vi "Offset Locking and Active Slave Locking v3.1.vi"() -> ()   [LabVIEW 2018]
uses:
  <vilib>/Utility/error.llb/DialogType.ctl
  <vilib>/Analysis/1siggen.llb/Ramp Pattern by Samples.vi
  <vilib>/measure/mamon.llb/Waveform Peak Detection for 1 Chan.vi
  <vilib>/addons/control/pid/pid.llb/PID Advanced (DBL).vi
  <vilib>/measure/NI_MAPro.lvlib
  <vilib>/addons/control/pid/NI_PID_pid.lvlib
  <vilib>/Analysis/NI_AALBase.lvlib
  <vilib>/measure/NI_MABase.lvlib
panel:
  out "Master-Slave Peak Height":dbl
  in  "Locked Peak Height Min":dbl
  in  "Active Slave Lock On":bool
  in  "Slave Current Adjust":dbl
  out "Target \nPeak":dbl
  out "Calibration\n Peaks":dbl[](array[numeric])
  in  "Minimum \namplitude\nfor Calibration":dbl=2.1 format="%#_13g V"
  in  "width":i32=1000
  in  "start":dbl format="%0.2f"
  in  "end":dbl=1.0 format="%0.2f"
  in  "samples":i32=128
  in  "Waveform Test?":bool
  in  "reset signal":bool
  in  "phase":dbl format="%.2p"
  out "Chirp Rate":dbl format="%#_g GHz/ms"
  out "Single Mode?":bool
  out "# of Peaks found when Chirping?":i32
  in  "Minimum amplitude for Slave":dbl=0.15 format="%.2p"
  in  "Minimum \namplitude\nfor peaks":dbl=1.2 format="%#_13g V"
  in  "PZT Voltage to \nFrequency Conversion":dbl=-1.41655 format="%#_g V/GHz"
  out "PZT Chirp Output":waveform(dbl)(graph)
  in  "offset":dbl format="%0.2p V"
  in  "Sampling Info":cluster{"Fs":dbl, "#s":dbl}={"Fs"=10000.0, "#s"=100.0} {"Fs" format="%.2p"}
  in  "frequency":dbl=10.0 format="%0.2p Hz"
  in  "Chirp Amplitude":dbl=1.5 format="%0.2p GHz"
  in  "Run Chirp Program?":bool
  out "Run Time (min)":dbl
  out "standard deviation":dbl format="%0.3e"
  out "# found":i32
  out "Offset":dbl(graph)
  in  "Manual PZT Control":dbl format="%#_g V"
  in  "Engage PZT PID?":bool
  out "Offset (GHz)":dbl format="%#_4g"
  in  "# of Shots for Averaging":i32=100
  in  "Name Convention":string="Chirp Offset Lock Log"
  in  "Save Directory":path=path "C:/Users/LabUser/Google Drive/Measurements/04-2018"
  out "Enough\n peaks?":bool
  out "PZT Output":dbl(graph)
  in  "PID Gains":T1={"proportional gain (Kc)"=-1.0, "integral time (Ti, min)"=0.01, "derivative time (Td, min)"=0.0} {"derivative time (Td, min)" format="%.3f"; "integral time (Ti, min)" format="%.3f"; "proportional gain (Kc)" format="%.3f"}
  out "dt out (s)":dbl format="%.3f"
  in  "Frequency Offset Setpoint (GHz)":dbl=4.0 format="%.3f"
  out "GHz/sec":dbl
  out "dt":dbl format="%#_4g"
  out "Locations":dbl[](array[numeric]) format="%.2p"
  out "Amplitudes":dbl[](array[numeric]) format="%.2p"
  out "2nd Derivatives":dbl[](array[numeric]) format="%.2p"
  out "10 GHz FPI":dynamicdata(graph)
  in  "Stop":bool
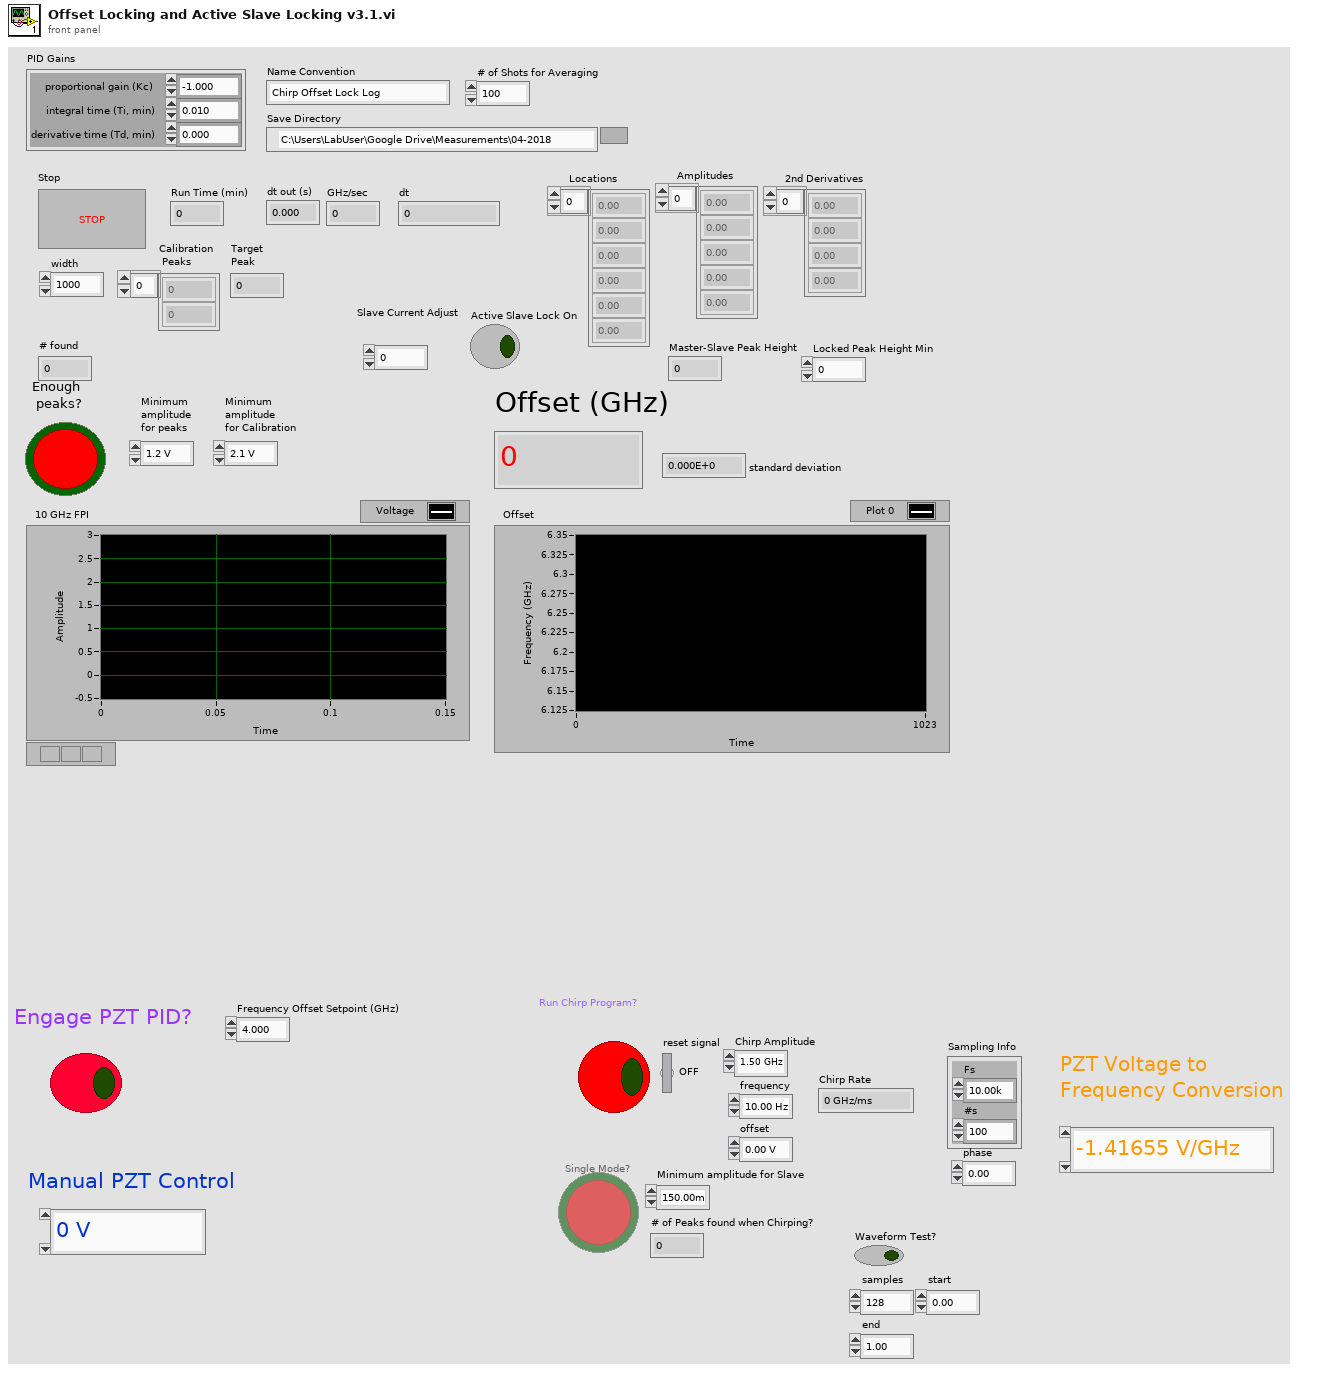
[diagram p1: front panel]
types:
  T1 = cluster{"proportional gain (Kc)":dbl, "integral time (Ti, min)":dbl, "derivative time (Td, min)":dbl}
  T2 = enum8{"Enabled", "Disabled", "Disabled and Grayed Out"}
  T3 = typedef "DialogType.ctl" = u16
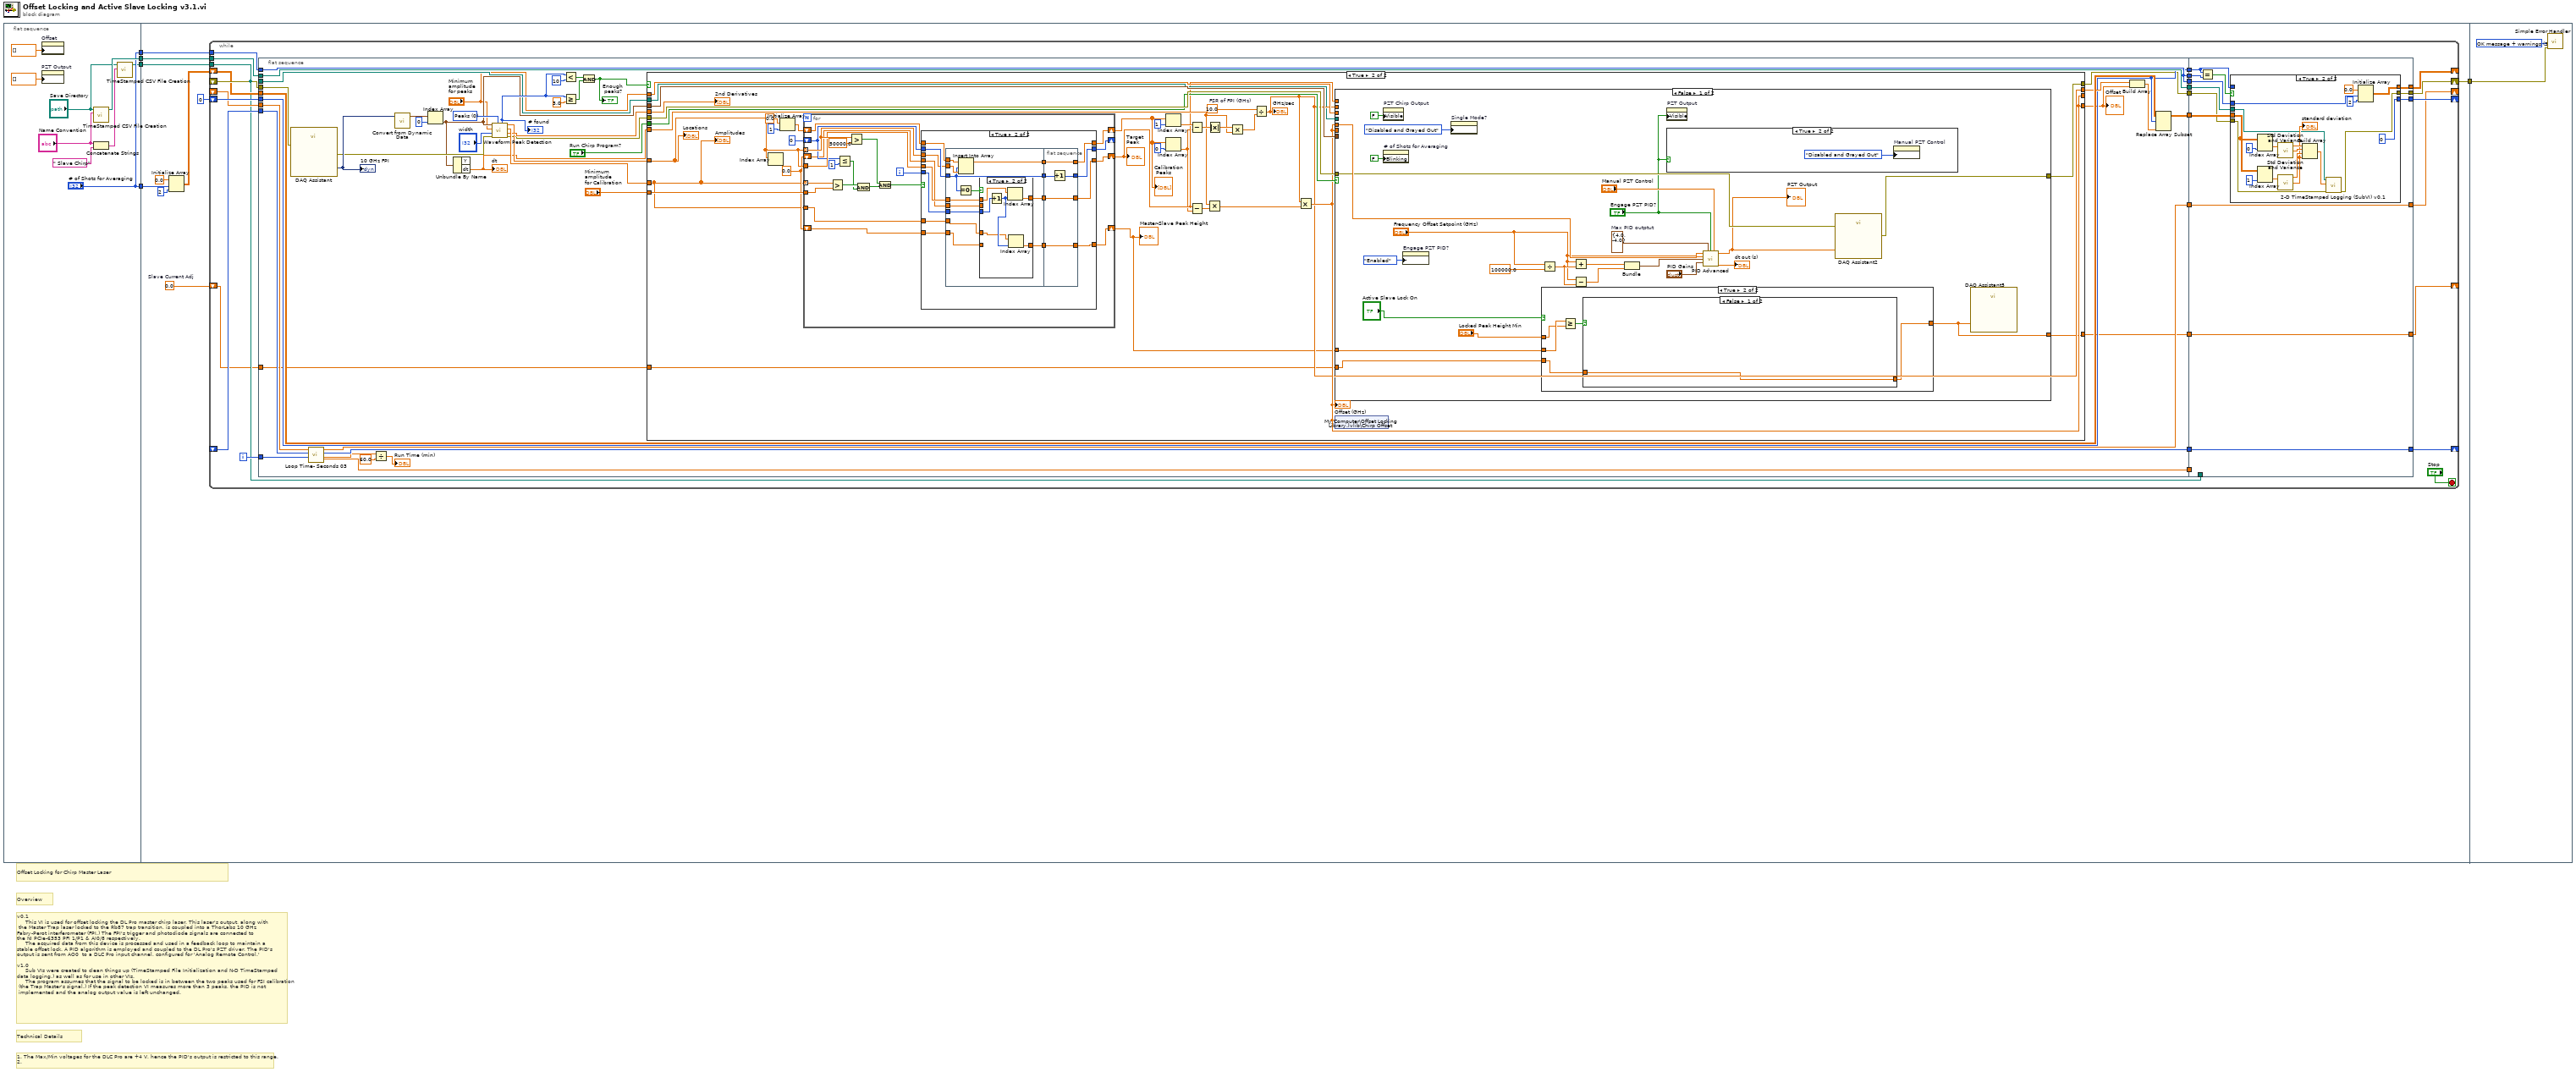
[diagram p0: block diagram]
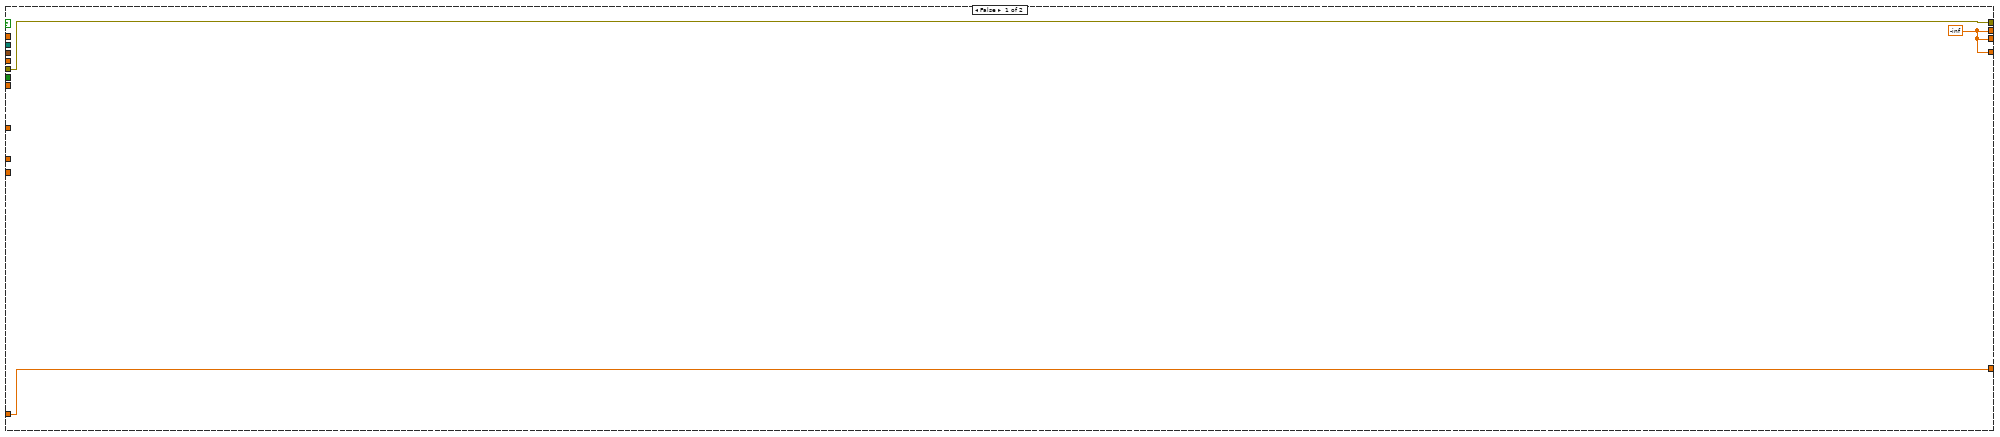
[diagram p2: hidden frame]
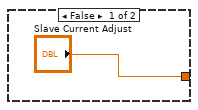
[diagram p5: hidden frame]
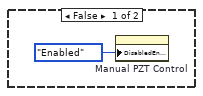
[diagram p7: hidden frame]
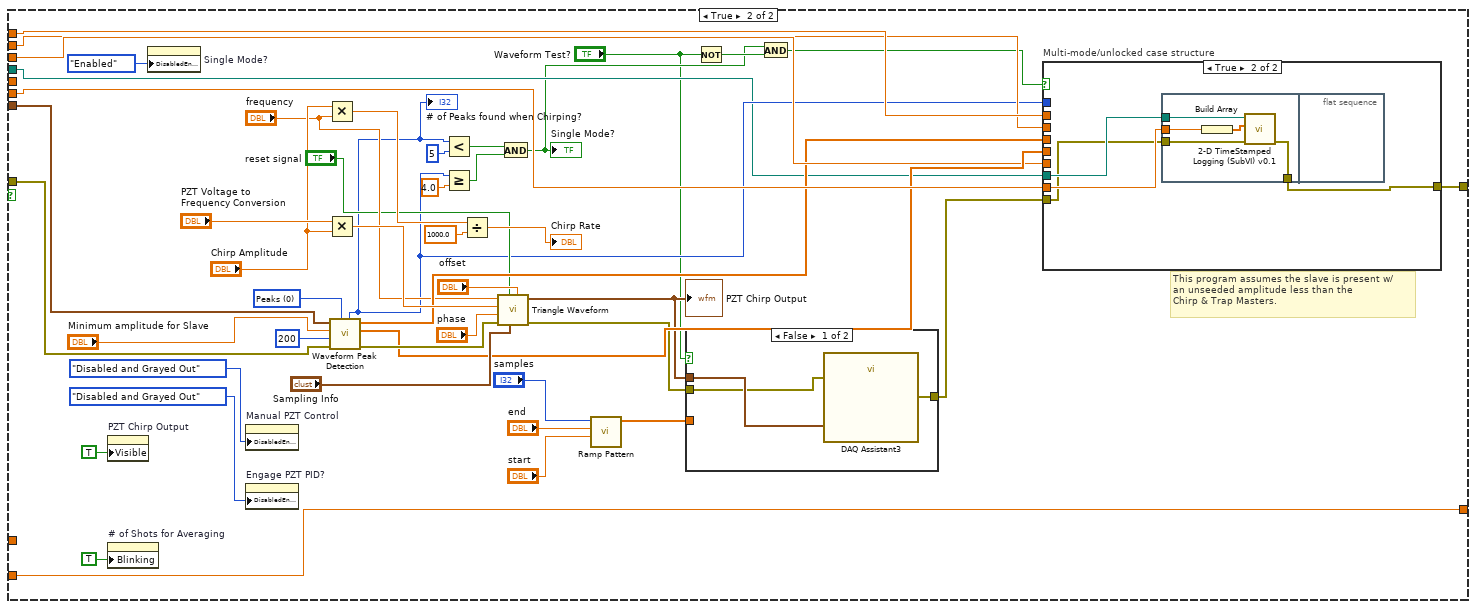
[diagram p8: hidden frame]
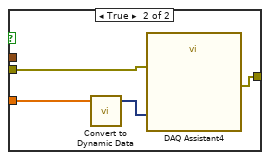
[diagram p9: hidden frame]
diagram:
  # "1. The Max/Min voltages for the DLC Pro are +4 V, hence the PID's output is restricted to this range.\n2."
  # "Technical Details"
  # "v0.1\n     This VI is used for offset locking the DL Pro master chirp laser. This laser's output, along with\n the Master Trap laser locked to the Rb87 trap transition, is coupled into a ThorLabs 10 GHz \nFabry-Perot interferometer (FPI.) The FPI's trigger and photodiode signals are connected to \nthe NI PCIe-6353 PFI 1/P1 & AI0/8 respectively. \n     The acquired data from this device is processed and used in a feedback loop to maintain a \nstable offset lock. A PID algorithm is employed and coupled to the DL Pro's PZT driver. The PID's\noutput is sent from AO0  to a DLC Pro input channel, configured for 'Analog Remote Control.'\n\nv1.0\n     Sub VIs were created to clean things up (TimeStamped File Initialization and N-D TimeStamped \ndata logging,) as well as for use in other VIs.\n     The program assumes that the signal to be locked is in between the two peaks used for FSI calibration\n (the Trap Master's signal.) If the peak detection VI measures more than 3 peaks, the PID is not\n implemented and the analog output value is left unchanged."
  # "Overview"
  # "Offset Locking for Chirp Master Laser"
  n1 = flat-sequence {
    tunnel: [w14] -> w5
    tunnel: ["# of Shots for Averaging"] -> w3
    tunnel: ["# of Shots for Averaging"] -> w2
    tunnel: [w6] -> w1
    tunnel: w5 -> [w24]
    tunnel: [w23] -> w4
    tunnel: w3 -> [w21]
    tunnel: w2 -> [w18]
    tunnel: w1 -> [w16]
    tunnel: w4 -> [w334]
    frame #0 {
      n2 = property on="Offset" class="WFChart (strict)"("History Data"=dbl[] []) -> ()  [unwired: 2 in, 2 out]
      n3 = property on="PZT Output" class="WFChart (strict)"("History Data"=dbl[] []) -> ()  [unwired: 2 in, 2 out]
      n4 = call "TimeStamped CSV File Creation.vi"("Name Convention"="Name Convention", "Save Directory"="Save Directory") -> ("path"=w14:path)  [unwired: 8 in, 1 out]
      n5 = Concatenate Strings("Name Convention", " Slave Chirp" ("string")) -> (w8:string)
      n6 = call "TimeStamped CSV File Creation.vi"("Name Convention"=w8, "Save Directory"="Save Directory") -> ("path"=w6:path)  [unwired: 8 in, 1 out]
    }
    frame #1 {
      w15 = 0.0  # Slave Current Adj
      n7 = Initialize Array(0.0 ("element"), w18, 2 ("dimension size")) -> (w20:dbl[][])
      n8 = while {
        shift-right: [w39] -> w23
        shift-left: _ -> [w50]
        tunnel: w24 -> [w48]
        shift-right: [w37] -> _
        shift-left: 0 -> [w46]
        tunnel: w21 -> [w44]
        shift-right: [w38] -> _
        shift-left: w20 -> [w41]
        shift-right: [w35] -> _
        shift-left: _ -> [w32]
        shift-right: [w33] -> _
        shift-left: _ -> [w31]
        tunnel: w16 -> [w28]
        shift-right: [w25] -> _
        shift-left: w15 -> [w27]
        i -> [w30]
        stop <- "Stop" stop-if-true
        n9 = flat-sequence {
          tunnel: w50 -> [w84]
          tunnel: [w60] -> w49
          tunnel: w48 -> [w82]
          tunnel: [w82] -> w47
          tunnel: w46 -> [w76]
          tunnel: [w76] -> w45
          tunnel: w44 -> [w77]
          tunnel: [w77] -> w43
          tunnel: [w81] -> w42
          tunnel: w41 -> [w80]
          tunnel: [w77] -> w40
          tunnel: [w75] -> w36
          tunnel: [w74] -> w34
          tunnel: w32 -> [w73]
          tunnel: w31 -> [w72]
          tunnel: w30 -> [w71]
          tunnel: [w63] -> w29
          tunnel: w28 -> [w57]
          tunnel: w27 -> [w53]
          tunnel: [w52] -> w26
          tunnel: w49 -> [w307]
          tunnel: w47 -> [w308]
          tunnel: w45 -> [w302]
          tunnel: w43 -> [w312]
          tunnel: w42 -> [w309]
          tunnel: w40 -> [w310]
          tunnel: [w301] -> w39
          tunnel: [w306] -> w38
          tunnel: [w305] -> w37
          tunnel: w36 -> [w304]
          tunnel: [w304] -> w35
          tunnel: [w303] -> w33
          tunnel: w34 -> [w303]
          tunnel: w29 -> [_]
          tunnel: w28 -> [_]
          tunnel: w26 -> [w300]
          tunnel: [w300] -> w25
          frame #0 {
            w86 = u16 0 items=["Peaks", "Valleys"] ("peaks/valleys")
            n10 = call "DAQ Assistant"("error in"=w84) -> ("data"=w91:dynamicdata, "error out"=w83:errorcluster)  [unwired: 16 in, 1 out]
            "10 GHz FPI" <- w91
            n11 = call "Loop Time- Seconds 03.vi"("Loop Iteration"=w71, "Shift Registered Time In"=w72, "Shift Registered In"=w73) -> ("t"=w63:dbl, "Shift Registered Time Out"=w74:u32, "Shift Registered Out"=w75:dbl)  [unwired: 6 in]
            n12 = Divide(x=w63, y=60.0) -> (x/y=→"Run Time (min)":dbl)
            n13 = call "Convert from Dynamic Data"("Dynamic Data Type"=w91) -> ("Array of Waveform"=w93:waveform(dbl)[])  [unwired: 3 in]
            n14 = Index Array(array=w93, index=0) -> (element=w58:waveform(dbl))
            n15 = Unbundle By Name(w58) -> ("dt"=w87:dbl)  [unwired: 1 out]
            "dt" <- w87
            n16 = call-poly <vilib>:"Waveform Peak Detection.vi"("peaks/valleys"=w86, "error in"=w83, "width"="width", "threshold"="Minimum \namplitude\nfor peaks", "Signal In"=w58) -> ("error out"=w61:errorcluster, "2nd Derivatives"=w89:dbl[], "Amplitudes"=w90:dbl[], "Locations"=w88:dbl[], "# found"=w68:i32)  [unwired: 2 in]
            "# found" <- w68
            n17 = Less?(x=w68, y=10) -> (x < y?=w66:bool)
            n18 = Greater Or Equal?(x=w68, y=3.0) -> (x >= y?=w69:bool)
            n19 = And(x=w66, y=w69) -> (x .and. y?=w65:bool)
            "Enough\n peaks?" <- w65
            n20 = case shown="True" w65 {
              tunnel: w90 -> [_ w100]
              tunnel: w89 -> [_ w129]
              tunnel: w88 -> [_ w108]
              tunnel: w87 -> [_ w123]
              tunnel: [w96 w115] -> w79
              tunnel: [w96 w117] -> w70
              tunnel: [w96 w117] -> _
              tunnel: w61 -> [w95 w121]
              tunnel: [w95 w120] -> w60
              tunnel: "Run Chirp Program?" -> [_ w119]
              tunnel: w58 -> [_ w118]
              tunnel: "Minimum \namplitude\nfor peaks" -> [_ w116]
              tunnel: w57 -> [_ w114]
              tunnel: "Minimum \namplitude\nfor Calibration" -> [_ w113]
              tunnel: w53 -> [w94 w98]
              tunnel: [w94 w97] -> w52
              frame False {
                w96 = -inf
              }
              frame True {
                w101 = 0.0
                w128 = 10.0  # FSR of FPI (GHz)
                n21 = Index Array(array=w108) -> ()  [unwired: 1 in, 1 out]
                n22 = Initialize Array(0.0 ("element"), 1 ("dimension size")) -> (w109:dbl[])
                n23 = for {
                  tunnel: w108 -> [w140] mode=indexing
                  tunnel: w100 -> [w133] mode=indexing
                  tunnel: w113 -> [w145]
                  shift-right: [w136] -> w107
                  shift-left: w109 -> [w150]
                  shift-right: [w149] -> _
                  shift-left: 0 -> [w137]
                  shift-right: [w135] -> w103
                  shift-left: w101 -> [w134]
                  tunnel: w108 -> [w138]
                  shift-right: [w131] -> w99
                  shift-left: w101 -> [w132]
                  tunnel: w100 -> [w130]
                  i -> [w139]
                  n24 = Greater?(x=w133, y=w145) -> (0:w148:bool)
                  n25 = Less Or Equal?(x=w137, y=1) -> (x <= y?=w146:bool)
                  n26 = Greater?(x=w140, y=50000.0) -> (0:w143:bool)
                  n27 = And(x=w148, y=w146) -> (x .and. y?=w144:bool)
                  n28 = And(x=w143, y=w144) -> (x .and. y?=w141:bool)
                  n29 = case shown="True" w141 {
                    tunnel: w150 -> [w153 w170]
                    tunnel: w137 -> [w154 w169]
                    tunnel: [w154 w166] -> w149
                    tunnel: w140 -> [_ w168]
                    tunnel: w139 -> [_ w163]
                    tunnel: w138 -> [_ w162]
                    tunnel: [w153 w164] -> w136
                    tunnel: [w152 w160] -> w135
                    tunnel: w134 -> [w152 w159]
                    tunnel: w132 -> [w151 w158]
                    tunnel: [w151 w155] -> w131
                    tunnel: w130 -> [_ w157]
                    frame False {
                    }
                    frame True {
                      n30 = flat-sequence {
                        tunnel: w170 -> [w182]
                        tunnel: w169 -> [w179]
                        tunnel: w168 -> [w181]
                        tunnel: [w180] -> w167
                        tunnel: [w179] -> w165
                        tunnel: w163 -> [w176]
                        tunnel: w162 -> [w178]
                        tunnel: [w177] -> w161
                        tunnel: w159 -> [w174]
                        tunnel: w158 -> [w171]
                        tunnel: w157 -> [w173]
                        tunnel: [w172] -> w156
                        tunnel: w167 -> [w193]
                        tunnel: [w195] -> w166
                        tunnel: w165 -> [w194]
                        tunnel: [w193] -> w164
                        tunnel: w161 -> [w192]
                        tunnel: [w192] -> w160
                        tunnel: w156 -> [w191]
                        tunnel: [w191] -> w155
                        frame #0 {
                          n31 = Equal To 0?(x=w179) -> (x = 0?=w175:bool)
                          n32 = Insert Into Array(array=w182, index=w179, new element=w181) -> (w180:dbl[])
                          n33 = case shown="True" w175 {
                            tunnel: w178 -> [_ w190]
                            tunnel: [w184 w189] -> w177
                            tunnel: w176 -> [_ w188]
                            tunnel: w174 -> [w184 _]
                            tunnel: w173 -> [_ w186]
                            tunnel: [w183 w185] -> w172
                            tunnel: w171 -> [w183 _]
                            frame False {
                            }
                            frame True {
                              n34 = Increment(x=w188) -> (x+1=w187:i32)
                              n35 = Index Array(array=w190, index=w187) -> (element=w189:dbl)
                              n36 = Index Array(array=w186, index=w187) -> (element=w185:dbl)
                            }
                          }
                        }
                        frame #1 {
                          n37 = Increment(x=w194) -> (x+1=w195:i32)
                        }
                      }
                    }
                  }
                }
                "Calibration\n Peaks" <- w107
                "Target \nPeak" <- w103
                "Master-Slave Peak Height" <- w99
                n38 = Index Array(array=w107, index=1) -> (element=w104:dbl)
                n39 = Index Array(array=w107, index=0) -> (element=w102:dbl)
                n40 = Subtract(x=w104, y=w102) -> (x-y=w126:dbl)
                n41 = Subtract(x=w103, y=w102) -> (x-y=w124:dbl)
                n42 = Multiply(x=w123, y=w124) -> (x*y=w122:dbl)
                n43 = Absolute Value(x=w126) -> (abs(x)=w125:dbl)
                n44 = Multiply(x=w125, y=w123) -> (x*y=w127:dbl)
                n45 = Divide(x=w128, y=w127) -> (x/y=w115:dbl)
                "GHz/sec" <- w115
                n46 = Multiply(x=w115, y=w122) -> (x*y=w117:dbl)
                "Offset (GHz)" <- w117
                n47 = case shown="False" w119 {
                  tunnel: w117 -> [w215 _]
                  tunnel: w121 -> [w214 w266]
                  tunnel: [w213 w239] -> w120
                  tunnel: w118 -> [_ w267]
                  tunnel: w117 -> [_ w263]
                  tunnel: w116 -> [_ w257]
                  tunnel: w103 -> [_ w255]
                  tunnel: w115 -> [_ w254]
                  tunnel: w114 -> [_ w241]
                  tunnel: w99 -> [w198 _]
                  tunnel: w98 -> [w197 w230]
                  tunnel: [w196 w230] -> w97
                  frame False {
                    w217 = cluster{"output high":dbl, "output low":dbl} {"output high"=4.0, "output low"=-4.0}  # Max PID outptut
                    n48 = property on="PZT Chirp Output" class="WFGraph (strict)"("Visible"=FALSE) -> ()  [unwired: 2 in, 2 out]
                    n49 = property on="# of Shots for Averaging" class="DigNum (strict)"("Blinking"=FALSE) -> ()  [unwired: 2 in, 2 out]
                    n50 = property on="Engage PZT PID?" class="Bool (strict)"("DisabledEnum"=T2."Enabled" ("Disabled")) -> ()  [unwired: 2 in, 2 out]
                    n51 = property on="Single Mode?" class="Bool (strict)"("DisabledEnum"=T2."Disabled and Grayed Out" ("Disabled")) -> ()  [unwired: 2 in, 2 out]
                    n52 = case shown="True" "Active Slave Lock On" {
                      tunnel: ["Slave Current Adjust" w221] -> w196
                      tunnel: "Locked Peak Height Min" -> [_ w223]
                      tunnel: w198 -> [_ w224]
                      tunnel: w197 -> [_ w222]
                      frame False {
                      }
                      frame True {
                        n53 = Greater Or Equal?(x=w224, y=w223) -> (x >= y?=w225:bool)
                        n54 = case shown="False" w225 {
                          tunnel: w222 -> [w226 w227]
                          tunnel: [w226 w227] -> w221
                          frame False {
                          }
                          frame True {
                          }
                        }
                      }
                    }
                    n55 = Divide(x="Frequency Offset Setpoint (GHz)", y=100000.0) -> (x/y=w205:dbl)
                    n56 = Add(x="Frequency Offset Setpoint (GHz)", y=w205) -> (x+y=w203:dbl)
                    n57 = Subtract(x="Frequency Offset Setpoint (GHz)", y=w205) -> (x-y=w202:dbl)
                    n58 = Bundle(w203, w202) -> (w201:cluster{dbl, dbl})  [unwired: 1 in]
                    n59 = property on="PZT Output" class="WFChart (strict)"("Visible"="Engage PZT PID?") -> ()  [unwired: 2 in, 2 out]
                    n60 = case shown="True" "Engage PZT PID?" {
                      frame False {
                        n61 = property on="Manual PZT Control" class="DigNum (strict)"("DisabledEnum"=T2."Enabled" ("Disabled")) -> ()  [unwired: 2 in, 2 out]
                      }
                      frame True {
                        n62 = property on="Manual PZT Control" class="DigNum (strict)"("DisabledEnum"=T2."Disabled and Grayed Out" ("Disabled")) -> ()  [unwired: 2 in, 2 out]
                      }
                    }
                    n63 = call-poly <vilib>:"PID Advanced.vi"("setpoint"="Frequency Offset Setpoint (GHz)", "output range"=w217, "auto? (T)"="Engage PZT PID?", "manual control"="Manual PZT Control", "process variable"=w215, "setpoint range"=w201, "PID gains"="PID Gains") -> ("output"=w212:dbl, "dt out (s)"=→"dt out (s)":dbl)  [unwired: 7 in]
                    "PZT Output" <- w212
                    n64 = call "DAQ Assistant2"("data"=w212, "error in"=w214) -> ("error out"=w213:errorcluster)  [unwired: 16 in, 1 out]
                    n65 = call "DAQ Assistant5"("data"=w196) -> ()  [unwired: 17 in, 2 out]
                  }
                  frame True {
                    w253 = u16 0 items=["Peaks", "Valleys"] ("peaks/valleys")
                    # "This program assumes the slave is present w/ \nan unseeded amplitude less than the \nChirp & Trap Masters."
                    n66 = property on="PZT Chirp Output" class="WFGraph (strict)"("Visible"=TRUE) -> ()  [unwired: 2 in, 2 out]
                    n67 = property on="# of Shots for Averaging" class="DigNum (strict)"("Blinking"=TRUE) -> ()  [unwired: 2 in, 2 out]
                    n68 = property on="Single Mode?" class="Bool (strict)"("DisabledEnum"=T2."Enabled" ("Disabled")) -> ()  [unwired: 2 in, 2 out]
                    n69 = property on="Manual PZT Control" class="DigNum (strict)"("DisabledEnum"=T2."Disabled and Grayed Out" ("Disabled")) -> ()  [unwired: 2 in, 2 out]
                    n70 = property on="Engage PZT PID?" class="Bool (strict)"("DisabledEnum"=T2."Disabled and Grayed Out" ("Disabled")) -> ()  [unwired: 2 in, 2 out]
                    n71 = Multiply(x="Chirp Amplitude", y="frequency") -> (x*y=w248:dbl)
                    n72 = Multiply(x="PZT Voltage to \nFrequency Conversion", y="Chirp Amplitude") -> (x*y=w269:dbl)
                    n73 = call-poly <vilib>:"Waveform Peak Detection.vi"("peaks/valleys"=w253, "error in"=w266, "width"=200, "threshold"="Minimum amplitude for Slave", "Signal In"=w267) -> ("error out"=w265:errorcluster, "Amplitudes"=w258:dbl[], "Locations"=w256:dbl[], "# found"=w242:i32)  [unwired: 2 in, 1 out]
                    "# of Peaks found when Chirping?" <- w242
                    n74 = Less?(x=w242, y=5) -> (x < y?=w259:bool)
                    n75 = Greater Or Equal?(x=w242, y=4.0) -> (x >= y?=w261:bool)
                    n76 = Divide(x=w248, y=1000.0) -> (x/y=→"Chirp Rate":dbl)
                    n77 = call <vilib>:"Triangle Waveform.vi"("offset"="offset", "sampling info"="Sampling Info", "reset signal"="reset signal", "error in (no error)"=w265, "phase"="phase", "amplitude"=w269, "frequency"="frequency") -> ("error out"=w243:errorcluster, "signal out"=w244:waveform(dbl))  [unwired: 3 in]
                    "PZT Chirp Output" <- w244
                    n78 = And(x=w259, y=w261) -> (x .and. y?=w237:bool)
                    "Single Mode?" <- w237
                    n79 = call-poly <vilib>:"Ramp Pattern.vi"("start"="start", "end"="end", "samples"="samples") -> ("Ramp Pattern"=w234:dbl[])  [unwired: 7 in, 1 out]
                    n80 = case shown="False" "Waveform Test?" {
                      tunnel: w244 -> [w279 _]
                      tunnel: w243 -> [w278 w283]
                      tunnel: [w277 w282] -> w240
                      tunnel: w234 -> [_ w281]
                      frame False {
                        n81 = call "DAQ Assistant3"("data"=w279, "error in"=w278) -> ("error out"=w277:errorcluster)  [unwired: 16 in, 1 out]
                      }
                      frame True {
                        n82 = call "Convert to Dynamic Data"("Array"=w281) -> ("Dynamic Data Type"=w280:dynamicdata)  [unwired: 3 in]
                        n83 = call "DAQ Assistant4"("data"=w280, "error in"=w283) -> ("error out"=w282:errorcluster)  [unwired: 16 in, 1 out]
                      }
                    }
                    n84 = Not(x="Waveform Test?") -> (.not. x?=w238:bool)
                    n85 = And(x=w237, y=w238) -> (x .and. y?=w236:bool)
                    n86 = case "Multi-mode/unlocked case structure" shown="True" w236 {
                      tunnel: w263 -> [_ w294]
                      tunnel: w242 -> [w290 _]
                      tunnel: w258 -> [w289 _]
                      tunnel: w257 -> [w288 _]
                      tunnel: w256 -> [w287 _]
                      tunnel: w255 -> [w286 _]
                      tunnel: w254 -> [w285 _]
                      tunnel: w241 -> [_ w293]
                      tunnel: w240 -> [w284 w292]
                      tunnel: [w284 w291] -> w239
                      frame False {
                        n87 = for {
                          N: w290 -> [_]
                          tunnel: w289 -> [_] mode=indexing
                          tunnel: w288 -> [_]
                          tunnel: w287 -> [_] mode=indexing
                          tunnel: w286 -> [_]
                          tunnel: w285 -> [_]
                        }
                      }
                      frame True {
                        n88 = flat-sequence {
                          tunnel: w294 -> [w299]
                          tunnel: w293 -> [w297]
                          tunnel: w292 -> [w296]
                          tunnel: [w295] -> w291
                          frame #0 {
                            n89 = Build Array(w299) -> (w298:dbl[])
                            n90 = call "2-D TimeStamped Logging (SubVI) v0.1.vi"("error in (no error)"=w296, "array"=w298, "path"=w297) -> ("error out"=w295:errorcluster)  [unwired: 8 in]
                          }
                          frame #1 {
                          }
                        }
                      }
                    }
                  }
                }
                n91 = shared-variable "My Computer\\Offset Locking Library.lvlib\\Chirp Offset"(w117) -> ()  [unwired: 1 in, 1 out]
                "2nd Derivatives" <- w129
                "Amplitudes" <- w100
                "Locations" <- w108
              }
            }
            "Offset" <- w70
            n92 = Build Array(w79, w70) -> (w78:dbl[])
            n93 = Replace Array Subset(array=w80, new element=w78, index (row)=w76) -> (w81:dbl[][])  [unwired: 1 in]
          }
          frame #1 {
            n94 = Equal?(x=w302, y=w312) -> (x = y?=w311:bool)
            n95 = case shown="True" w311 {
              tunnel: w310 -> [_ w316]
              tunnel: w309 -> [w315 w329]
              tunnel: w308 -> [_ w323]
              tunnel: w307 -> [w313 w322]
              tunnel: [w315 w319] -> w306
              tunnel: w302 -> [w314 _]
              tunnel: [w314 0] -> w305
              tunnel: [w313 w317] -> w301
              frame False {
              }
              frame True {
                n96 = Index Array(array=w329, index (col)=0 ("disabled index (col)")) -> (element=w332:dbl[])  [unwired: 1 in]
                n97 = Index Array(array=w329, index (col)=1 ("disabled index (col)")) -> (element=w330:dbl[])  [unwired: 1 in]
                n98 = call <vilib>:"Std Deviation and Variance.vi"("X"=w332) -> ("mean"=w328:dbl, "standard deviation"=w327:dbl)  [unwired: 1 in, 1 out]
                n99 = call <vilib>:"Std Deviation and Variance.vi"("X"=w330) -> ("mean"=w326:dbl, "standard deviation"=w325:dbl)  [unwired: 1 in, 1 out]
                "standard deviation" <- w325
                n100 = Build Array(w328, w327, w326, w325) -> (w324:dbl[])
                n101 = call "2-D TimeStamped Logging (SubVI) v0.1.vi"("error in (no error)"=w322, "array"=w324, "path"=w323) -> ("error out"=w317:errorcluster)  [unwired: 8 in]
                n102 = Initialize Array(0.0 ("element"), w316, 2 ("dimension size")) -> (w319:dbl[][])
              }
            }
          }
        }
      }
    }
    frame #2 {
      w335 = T3 3 items=["no dialog", "OK message", "continue or stop message", "OK message + warnings", "continue/stop + warnings"] ("type of dialog (OK msg:1)")
      n103 = call <vilib>:"Simple Error Handler.vi"("type of dialog (OK msg:1)"=w335, "error in (no error)"=w334) -> ()  [unwired: 3 in, 5 out]
    }
  }
